vi "Finish.vi"() -> ()   [LabVIEW 2017]
doc: "This VI is called just before exiting. It is expected to close I/O refnum, save collected data, etc."
uses:
  <vilib>/Rock Robotics/WPI/Utilities/WPI_GetSetVariantRefNum.vi
  <vilib>/Rock Robotics/WPI/Ultrasonic/WPI_SonarSRF04DigitalRefNum Registry Get.vi
  <vilib>/Rock Robotics/WPI/Ultrasonic/WPI_SonarSRF04DigitalClose.vi
panel:
  out "error out":errorcluster
  in  "error in":errorcluster
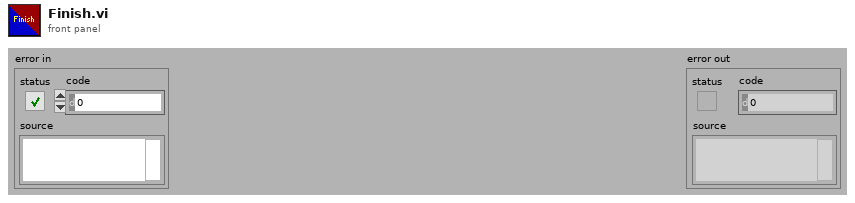
[diagram p1: front panel]
types:
  T1 = typedef "WPI_JoystickDevRef.ctl" = cluster{"Device":T2}
  T2 = typedef "WPI_JoystickDeviceEnum.ctl" = enum16{"USB 0", "USB 1", "USB 2", "USB 3", "USB 4", "USB 5"}
  T3 = typedef "WPI_RobotDriveDevRef.ctl" = cluster{"DevStatus":errorcluster, "Motors[]":T4[], "Square Inputs":bool, "Max Output":dbl}
  T4 = typedef "WPI_MotorControlDeviceRef.ctl" = cluster{"DeviceStatus":errorcluster, "Type":T5, "PWM":cluster{"PWM Channel":T6, "DeadBand":T7}, "CAN":cluster{"Device Number":u8, "SetOutput VI Ref":variant, "GetOutput VI Ref":variant, "Enable VI Ref":variant, "Disable VI Ref":variant, "Data":variant}, "Invert":bool, "DIO PWM":cluster{"PWM \"Enable\" Channel":T6, "DIOChannel":T8, "PWM Rate":dbl}}
  T5 = typedef "WPI_MotorControlType.ctl" = enum16{"PWM", "CAN", "DIO PWM"}
  T6 = typedef "FPGA_DIOPWMChannel.ctl" = enum8{"PWM 0", "PWM 1", "PWM 2", "PWM 3", "PWM 4", "PWM 5", "PWM 6", "PWM 7", "PWM 8", "PWM 9", "PWM MXP 0", "PWM MXP 1", "PWM MXP 2", "PWM MXP 3", "PWM MXP 4", "PWM MXP 5", "PWM MXP 6", "PWM MXP 7", "PWM MXP 8", "PWM MXP 9", "Invalid"}
  T7 = typedef "WPI_PWMDeadband.ctl" = cluster{"Name":string, "maxPositivePwm":i32, "minPositivePwm":i32, "centerPwm":i32, "maxNegativePwm":i32, "minNegativePwm":i32, "angularRange":u16}
  T8 = typedef "FPGA_DIOChannel.ctl" = enum8{"DIO 0", "DIO 1", "DIO 2", "DIO 3", "DIO 4", "DIO 5", "DIO 6", "DIO 7", "DIO 8", "DIO 9", "DIO MXP 0", "DIO MXP 1", "DIO MXP 2", "DIO MXP 3", "DIO MXP 4", "DIO MXP 5", "DIO MXP 6", "DIO MXP 7", "DIO MXP 8", "DIO MXP 9", "DIO MXP 10", "DIO MXP 11", "DIO MXP 12", "DIO MXP 13", "DIO MXP 14", "DIO MXP 15", "SPI Port CS1", "SPI Port CS2", "SPI Port CS3", "SPI Port MISO", "SPI Port MOSI", "Invalid"}
  T9 = typedef "WPI_GyroDevRef.ctl" = cluster{"DevStatus":errorcluster, "Analog Channel":T10, "Gain (VoltsPerDegree/Second)":dbl, "Gyro Type":enum16{"Analog", "XRS450"}, "Handle":i32, "SPI Bus":T11, "Device Found":bool, "Sample Rate":dbl, "Calibrate On Open":bool, "Offset":dbl}
  T10 = typedef "FPGA_AIChannel.ctl" = enum8{"AI 0", "AI 1", "AI 2", "AI 3", "AI MXP 0", "AI MXP 1", "AI MXP 2", "AI MXP 3", "Invalid"}
  T11 = typedef "spi_bus.ctl" = enum16{"SPI On-Board, CS0", "SPI On-Board, CS1", "SPI On-Board, CS2", "SPI On-Board, CS3", "SPI MXP", "Invalid"}
  T12 = typedef "WPI_SwitchDevRef.ctl" = cluster{"DevStatus":errorcluster, "DIO Channel":T8, "CntIndex":T13, "Normally Closed":bool}
  T13 = typedef "FPGA_CounterCtrSystemIndex.ctl" = enum8{"Ctr 0", "Ctr 1", "Ctr 2", "Ctr 3", "Ctr 4", "Ctr 5", "Ctr 6", "Ctr 7", "Invalid"}
  T14 = typedef "WPI_SolenoidDevRef.ctl" = cluster{"DevStatus":errorcluster, "Pneumatics Control Module":u8, "Forward Solenoid Channel":T15, "Reverse Solenoid Channel":T15}
  T15 = typedef "WPI_SolenoidChannel.ctl" = enum8{"Solenoid 0", "Solenoid 1", "Solenoid 2", "Solenoid 3", "Solenoid 4", "Solenoid 5", "Solenoid 6", "Solenoid 7", "Invalid"}
  T16 = typedef "WPI_CompressorDevRef.ctl" = cluster{"DevStatus":errorcluster, "Pneumatics Control Module":u8}
  T17 = typedef "WPI_AccelerometerDevRef.ctl" = cluster{"DevStatus":errorcluster, "Scaling":T18, "Analog Channels":T19, "I2C Bus":T20, "SPI Bus":T11, "Accel Range":T21, "ADXL Axes":T22, "Handle":i32, "Device Address":u8, "Accel Type":enum16{"Analog", "ADXL345 I2C", "ADXL345 SPI", "Internal", "ADXL362 SPI"}}
  T18 = typedef "WPI_AccelerometerScaling.ctl" = cluster{"Gain (VoltsPerG)":dbl, "Center Voltage":dbl}
  T19 = typedef "WPI_AccelerometerAnalogChannels.ctl" = cluster{"X-Axis":T10, "Y-Axis":T10, "Z-Axis":T10}
  T20 = typedef "i2c_bus.ctl" = enum16{"I2C On-Board", "I2C MXP", "Invalid"}
  T21 = typedef "ADXL345 Range.ctl" = u8
  T22 = typedef "WPI_AccelerometerADXL345 Axes.ctl" = cluster{"X-Axis":bool, "Y-Axis":bool, "Z-Axis":bool}
  T23 = typedef "WPI_UltrasonicDeviceRef.ctl" = cluster{"DevStatus":errorcluster, "Ping Channel":T8, "Echo Channel":T8, "CntIndex":T13}
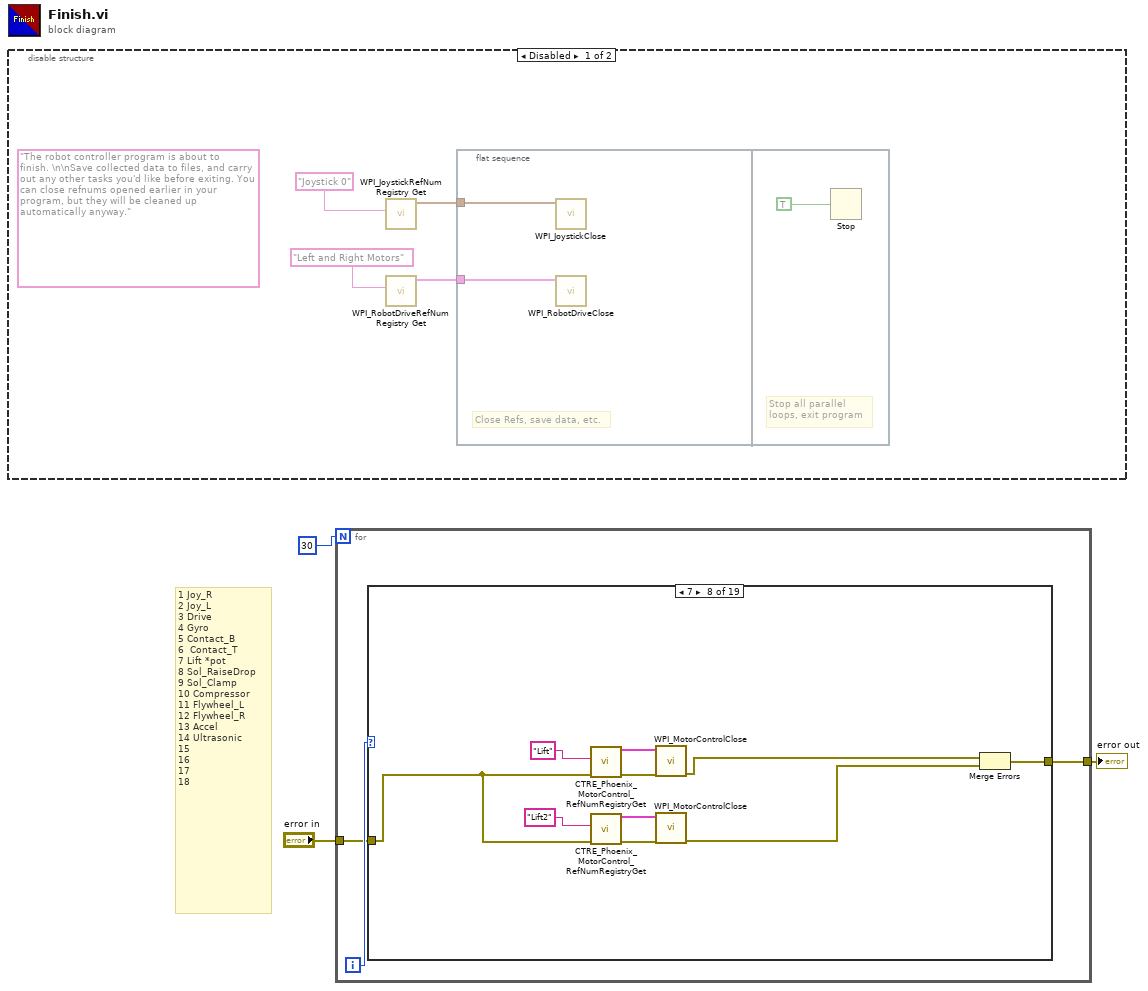
[diagram p0: block diagram]
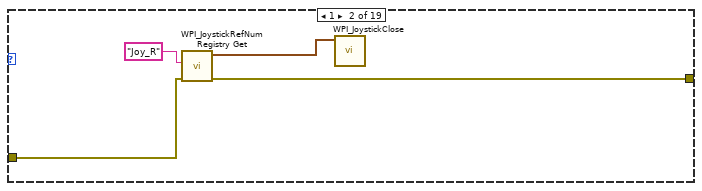
[diagram p3: hidden frame]
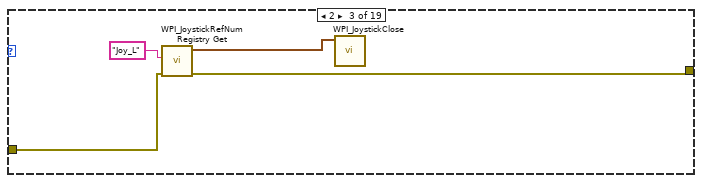
[diagram p4: hidden frame]
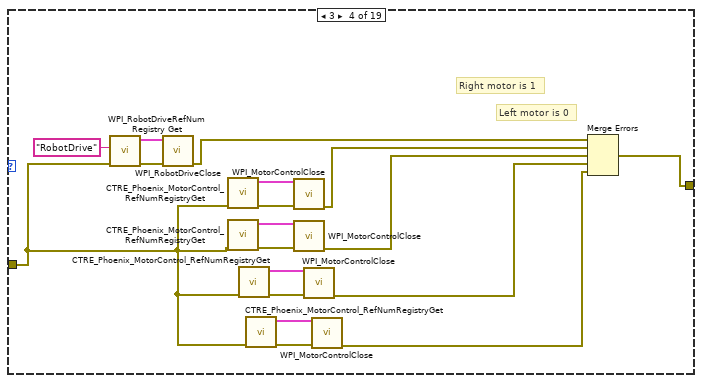
[diagram p5: hidden frame]
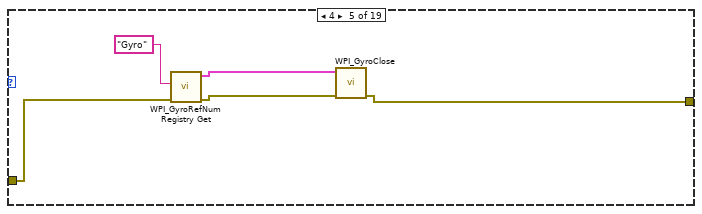
[diagram p6: hidden frame]
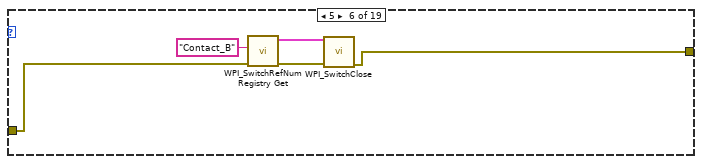
[diagram p7: hidden frame]
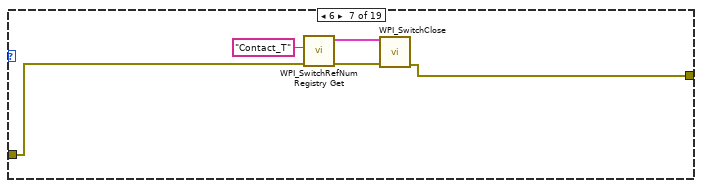
[diagram p8: hidden frame]
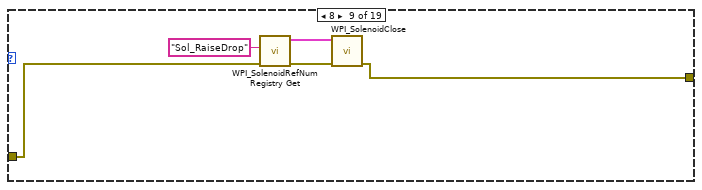
[diagram p9: hidden frame]
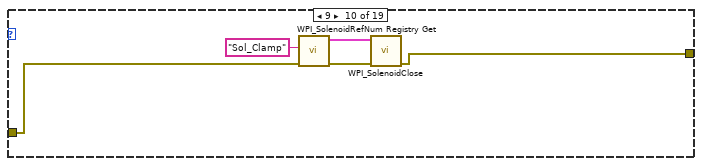
[diagram p10: hidden frame]
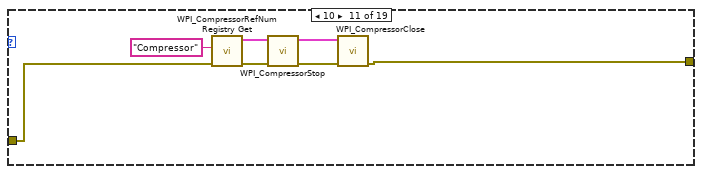
[diagram p11: hidden frame]
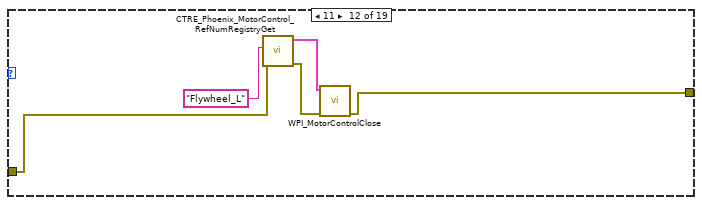
[diagram p12: hidden frame]
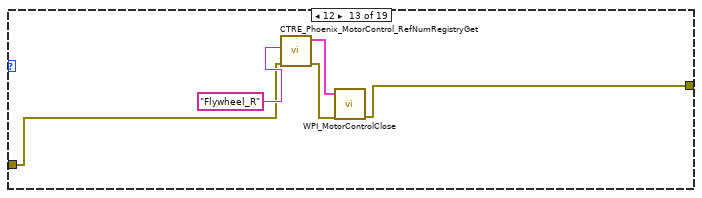
[diagram p13: hidden frame]
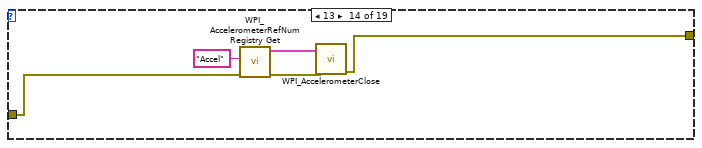
[diagram p14: hidden frame]
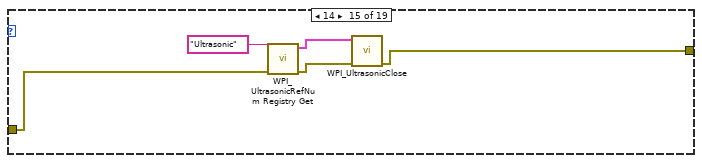
[diagram p15: hidden frame]
diagram:
  # "1 Joy_R\n2 Joy_L\n3 Drive\n4 Gyro\n5 Contact_B\n6  Contact_T\n7 Lift *pot\n8 Sol_RaiseDrop\n9 Sol_Clamp\n10 Compressor\n11 Flywheel_L\n12 Flywheel_R\n13 Accel\n14 Ultrasonic\n15\n16\n17\n18"
  n1 = disable-structure shown="Disabled" {
    frame Disabled {
      (unwired) "The robot controller program is about to finish. \n\nSave collected data to files, and carry out any other tasks you'd like before exiting. You can close refnums opened earlier in your program, but they will be cleaned up automatically anyway."
      n2 = call <vilib>:"WPI_JoystickRefNum Registry Get.vi"("refnum name"="Joystick 0") -> ("JoystickDevRef"=w4:T1)  [unwired: 1 in, 9 out]
      n3 = call <vilib>:"WPI_RobotDriveRefNum Registry Get.vi"("refnum name"="Left and Right Motors") -> ("RobotDriveDevRef"=w5:T3)  [unwired: 1 in, 9 out]
      n4 = flat-sequence {
        tunnel: w5 -> [w9]
        tunnel: w4 -> [w8]
        frame #0 {
          # "Close Refs, save data, etc."
          n5 = call <vilib>:"WPI_JoystickClose.vi"("JoystickDevRef"=w8) -> ()  [unwired: 11 out]
          n6 = call <vilib>:"WPI_RobotDriveClose.vi"("RobotDriveDevRef"=w9) -> ()  [unwired: 1 in, 10 out]
        }
        frame #1 {
          # "Stop all parallel\nloops, exit program"
          n7 = Stop(stop? (T)=TRUE ("Quit")) -> ()
        }
      }
    }
    frame Enabled {
    }
  }
  n8 = for {
    N: 30 -> [_]
    tunnel: "error in" -> [w12]
    tunnel: [w11] -> w1
    i -> [w13]
    n9 = case shown="7" w13 {
      tunnel: w12 -> [w14 w16 w20 w29 w44 w50 w52 w59 w70 w73 w77 w85 w90 w96 w102 w103 w104 w105 w106]
      tunnel: [w14 w15 w19 w24 w42 w48 w51 w58 w67 w71 w78 w87 w92 w94 w98 w103 w104 w105 w106] -> w11
      frame 0, Default {
      }
      frame 1 {
        n10 = call <vilib>:"WPI_JoystickRefNum Registry Get.vi"("error in (no error)"=w16, "refnum name"="Joy_R") -> ("error out"=w15:errorcluster, "JoystickDevRef"=w17:T1)  [unwired: 8 in]
        n11 = call <vilib>:"WPI_JoystickClose.vi"("JoystickDevRef"=w17) -> ()  [unwired: 11 in]
      }
      frame 2 {
        n12 = call <vilib>:"WPI_JoystickRefNum Registry Get.vi"("error in (no error)"=w20, "refnum name"="Joy_L") -> ("error out"=w19:errorcluster, "JoystickDevRef"=w21:T1)  [unwired: 8 in]
        n13 = call <vilib>:"WPI_JoystickClose.vi"("JoystickDevRef"=w21) -> ()  [unwired: 11 in]
      }
      frame 3 {
        # "Left motor is 0"
        # "Right motor is 1"
        n14 = call <vilib>:"WPI_RobotDriveRefNum Registry Get.vi"("error in (no error)"=w29, "refnum name"="RobotDrive") -> ("error out"=w40:errorcluster, "RobotDriveDevRef"=w38:T3)  [unwired: 8 in]
        n15 = call <vilib>:"WPI_RobotDriveClose.vi"("error in (no error)"=w40, "RobotDriveDevRef"=w38) -> ("error out"=w23:errorcluster)  [unwired: 9 in]
        n16 = call <vilib>:"CTRE_Phoenix_MotorControl_RefNumRegistryGet.vi"("error in (no error)"=w29) -> ("error out"=w32:errorcluster, "PhoenixMotorControlDevRef"=w33:T4)  [unwired: 9 in]
        n17 = call <vilib>:"CTRE_Phoenix_MotorControl_RefNumRegistryGet.vi"("error in (no error)"=w29) -> ("error out"=w36:errorcluster, "PhoenixMotorControlDevRef"=w37:T4)  [unwired: 9 in]
        n18 = call <vilib>:"CTRE_Phoenix_MotorControl_RefNumRegistryGet.vi"("error in (no error)"=w29) -> ("error out"=w34:errorcluster, "PhoenixMotorControlDevRef"=w35:T4)  [unwired: 9 in]
        n19 = call <vilib>:"CTRE_Phoenix_MotorControl_RefNumRegistryGet.vi"("error in (no error)"=w29) -> ("error out"=w30:errorcluster, "PhoenixMotorControlDevRef"=w31:T4)  [unwired: 9 in]
        n20 = call <vilib>:"WPI_MotorControlClose.vi"("error in"=w32, "MotorControlDevRef"=w33) -> ("error out"=w28:errorcluster)  [unwired: 9 in]
        n21 = call <vilib>:"WPI_MotorControlClose.vi"("error in"=w36, "MotorControlDevRef"=w37) -> ("error out"=w27:errorcluster)  [unwired: 9 in]
        n22 = call <vilib>:"WPI_MotorControlClose.vi"("error in"=w34, "MotorControlDevRef"=w35) -> ("error out"=w26:errorcluster)  [unwired: 9 in]
        n23 = call <vilib>:"WPI_MotorControlClose.vi"("error in"=w30, "MotorControlDevRef"=w31) -> ("error out"=w25:errorcluster)  [unwired: 9 in]
        n24 = Merge Errors(w23, w28, w27, w26, w25) -> (w24:errorcluster)
      }
      frame 4 {
        n25 = call <vilib>:"WPI_GyroRefNum Registry Get.vi"("error in (no error)"=w44, "refnum name"="Gyro") -> ("error out"=w43:errorcluster, "GyroDevRef"=w45:T9)  [unwired: 8 in]
        n26 = call <vilib>:"WPI_GyroClose.vi"("error in"=w43, "GyroDevRef"=w45) -> ("error out"=w42:errorcluster)  [unwired: 9 in]
      }
      frame 5 {
        n27 = call <vilib>:"WPI_SwitchRefNum Registry Get.vi"("error in (no error)"=w50, "refnum name"="Contact_B") -> ("error out"=w49:errorcluster, "SwitchDevRef"=w47:T12)  [unwired: 8 in]
        n28 = call <vilib>:"WPI_SwitchClose.vi"("error in (no error)"=w49, "SwitchDevRef"=w47) -> ("error out"=w48:errorcluster)  [unwired: 9 in]
      }
      frame 6 {
        n29 = call <vilib>:"WPI_SwitchRefNum Registry Get.vi"("error in (no error)"=w52, "refnum name"="Contact_T") -> ("error out"=w54:errorcluster, "SwitchDevRef"=w55:T12)  [unwired: 8 in]
        n30 = call <vilib>:"WPI_SwitchClose.vi"("error in (no error)"=w54, "SwitchDevRef"=w55) -> ("error out"=w51:errorcluster)  [unwired: 9 in]
      }
      frame 7 {
        n31 = call <vilib>:"CTRE_Phoenix_MotorControl_RefNumRegistryGet.vi"("error in (no error)"=w59, "refnum name"="Lift") -> ("error out"=w64:errorcluster, "PhoenixMotorControlDevRef"=w63:T4)  [unwired: 8 in]
        n32 = call <vilib>:"CTRE_Phoenix_MotorControl_RefNumRegistryGet.vi"("error in (no error)"=w59, "refnum name"="Lift2") -> ("error out"=w61:errorcluster, "PhoenixMotorControlDevRef"=w60:T4)  [unwired: 8 in]
        n33 = call <vilib>:"WPI_MotorControlClose.vi"("error in"=w64, "MotorControlDevRef"=w63) -> ("error out"=w57:errorcluster)  [unwired: 9 in]
        n34 = call <vilib>:"WPI_MotorControlClose.vi"("error in"=w61, "MotorControlDevRef"=w60) -> ("error out"=w56:errorcluster)  [unwired: 9 in]
        n35 = Merge Errors(w57, w56) -> (w58:errorcluster)
      }
      frame 8 {
        n36 = call <vilib>:"WPI_SolenoidRefNum Registry Get.vi"("error in (no error)"=w70, "refnum name"="Sol_RaiseDrop") -> ("error out"=w68:errorcluster, "SolenoidDevRef"=w69:T14)  [unwired: 8 in]
        n37 = call <vilib>:"WPI_SolenoidClose.vi"("error in (no error)"=w68, "SolenoidDevRef"=w69) -> ("error out"=w67:errorcluster)  [unwired: 9 in]
      }
      frame 9 {
        n38 = call <vilib>:"WPI_SolenoidRefNum Registry Get.vi"("error in (no error)"=w73, "refnum name"="Sol_Clamp") -> ("error out"=w72:errorcluster, "SolenoidDevRef"=w75:T14)  [unwired: 8 in]
        n39 = call <vilib>:"WPI_SolenoidClose.vi"("error in (no error)"=w72, "SolenoidDevRef"=w75) -> ("error out"=w71:errorcluster)  [unwired: 9 in]
      }
      frame 10 {
        n40 = call <vilib>:"WPI_CompressorRefNum Registry Get.vi"("error in (no error)"=w77, "refnum name"="Compressor") -> ("error out"=w81:errorcluster, "CompressorDevRef"=w82:T16)  [unwired: 8 in]
        n41 = call <vilib>:"WPI_CompressorStop.vi"("error in (no error)"=w81, "CompressorDevRef"=w82) -> ("error out"=w80:errorcluster, "CompressorDevRef"=w79:T16)  [unwired: 8 in]
        n42 = call <vilib>:"WPI_CompressorClose.vi"("error in (no error)"=w80, "CompressorDevRef"=w79) -> ("error out"=w78:errorcluster)  [unwired: 9 in]
      }
      frame 11 {
        n43 = call <vilib>:"CTRE_Phoenix_MotorControl_RefNumRegistryGet.vi"("error in (no error)"=w85, "refnum name"="Flywheel_L") -> ("error out"=w84:errorcluster, "PhoenixMotorControlDevRef"=w83:T4)  [unwired: 8 in]
        n44 = call <vilib>:"WPI_MotorControlClose.vi"("error in"=w84, "MotorControlDevRef"=w83) -> ("error out"=w87:errorcluster)  [unwired: 9 in]
      }
      frame 12 {
        n45 = call <vilib>:"CTRE_Phoenix_MotorControl_RefNumRegistryGet.vi"("error in (no error)"=w90, "refnum name"="Flywheel_R") -> ("error out"=w89:errorcluster, "PhoenixMotorControlDevRef"=w88:T4)  [unwired: 8 in]
        n46 = call <vilib>:"WPI_MotorControlClose.vi"("error in"=w89, "MotorControlDevRef"=w88) -> ("error out"=w92:errorcluster)  [unwired: 9 in]
      }
      frame 13 {
        n47 = call <vilib>:"WPI_AccelerometerRefNum Registry Get.vi"("error in (no error)"=w96, "refnum name"="Accel") -> ("error out"=w95:errorcluster, "AccelerometerDevRef"=w93:T17)  [unwired: 8 in]
        n48 = call <vilib>:"WPI_AccelerometerClose.vi"("error in"=w95, "AccelerometerDevRef"=w93) -> ("error out"=w94:errorcluster)  [unwired: 9 in]
      }
      frame 14 {
        n49 = call-poly <vilib>:"WPI_UltrasonicRefNum Registry Get.vi"("error in (no error)"=w102, "refnum name"="Ultrasonic") -> ("error out"=w100:errorcluster, "SonarSRF04DevRef"=w99:T23)  [unwired: 8 in]
        n50 = call-poly <vilib>:"WPI_UltrasonicClose.vi"("error in (no error)"=w100, "SonarSRF04DevRef"=w99) -> ("error out"=w98:errorcluster)  [unwired: 9 in]
      }
      frame 15 {
      }
      frame 16 {
      }
      frame 17 {
      }
      frame 18 {
      }
    }
  }
  "error out" <- w1
